vi "LVProjectShortcut_Item_CanDragToProjectWindow.vi"(10 "DropTarget":T1, 11 "Object":T1) -> (3 "CanDrag":bool)   [LabVIEW 2017, in "LVProject Shortcut.lvlib"]
uses:
  <resource>/Framework/Providers/API/ItemRef.ctl
  LVProject Shortcut.lvlib
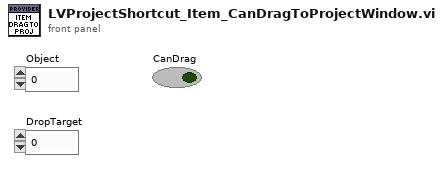
[diagram p1: front panel]
types:
  T1 = typedef "ItemRef.ctl" = u64
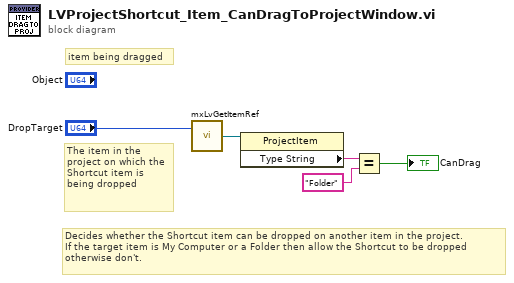
[diagram p0: block diagram]
diagram:
  # "item being dragged"
  # "Decides whether the Shortcut item can be dropped on another item in the project. \nIf the target item is My Computer or a Folder then allow the Shortcut to be dropped\notherwise don't."
  # "The item in the project on which the Shortcut item is being dropped"
  n1 = call <resource>:"mxLvGetItemRef.vi"("Item"="DropTarget") -> ("Item Refnum"=w4:refnum<vi>)  [unwired: 1 in, 2 out]
  n2 = property class="ProjectItem"(reference=w4) -> ("Type String"=w5:string)  [unwired: 1 in, 2 out]
  n3 = Equal?(x=w5, y="Folder" ("Type String")) -> (x = y?=→"CanDrag":bool)
